vi "VisitLVType.vi"(8 "error in (no error)":errorcluster, 10 "LVType":refnum<class "LVType.lvclass">, 11 "GetTypeAttributesVisitor in":refnum<class "GetTypeAttributesVisitor.lvclass">) -> (0 "error out":errorcluster, 3 "GetTypeAttributesVisitor out":refnum<class "GetTypeAttributesVisitor.lvclass">)   [LabVIEW 2020, in "Web Service Description.lvlib" / "GetTypeAttributesVisitor.lvclass"]
uses:
  <vilib>/AppBuilder/Engine/WebServiceDescription/GetTypeAttributesVisitor/GetTypeAttributesVisitor.lvclass
  <vilib>/AppBuilder/Engine/WebServiceDescription/LVDataTypes/LVType/LVType.lvclass
  <vilib>/AppBuilder/Engine/WebServiceDescription/GetTypeAttributesVisitor/GetTypeAttributesVisitor.lvclass/GetTypeAttributesVisitor.ctl
  <vilib>/AppBuilder/Engine/WebServiceDescription/XMLGen/ValuePair.ctl
  <vilib>/AppBuilder/Engine/WebServiceDescription/XMLGen/XMLGen.lvlib
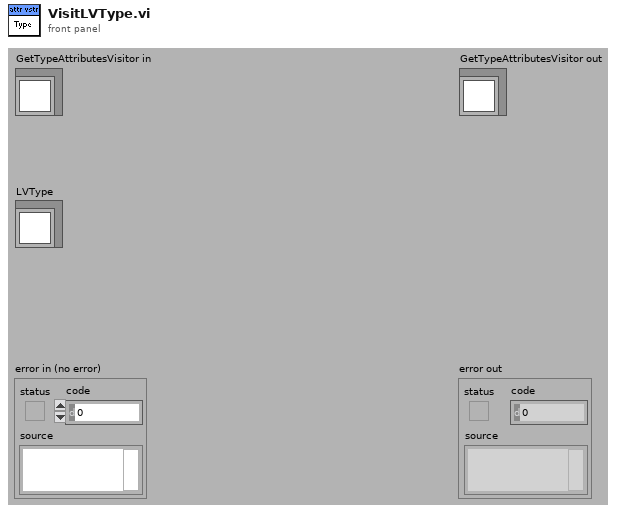
[diagram p1: front panel]
types:
  T1 = typedef "XMLGen.lvlib/ValuePair.ctl" = cluster{"Name":string, "Value":string}
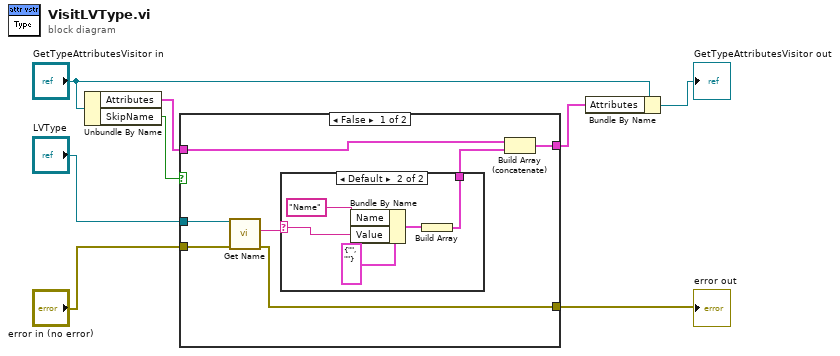
[diagram p0: block diagram]
diagram:
  n1 = Unbundle By Name("GetTypeAttributesVisitor in") -> ("Attributes"=w6:T1[], "SkipName"=w1:bool)
  n2 = case shown="False" w1 {
    tunnel: w6 -> [w15 w22]
    tunnel: "LVType" -> [w14 _]
    tunnel: "error in (no error)" -> [w13 w21]
    tunnel: [w12 w21] -> w3
    tunnel: [w11 w22] -> w2
    frame False {
      n3 = call <vilib>:"Get Name.vi"("error in (no error)"=w13, "LVType.lvclass in"=w14) -> ("error out"=w12:errorcluster, "Name"=w10:string)  [unwired: 8 out]
      n4 = case shown="Default" w10 {
        selector: w10 -> [_ w18]
        tunnel: [_ w16] -> w9
        frame "" {
        }
        frame Default {
          n5 = Bundle By Name(cluster=T1 {"Name"="", "Value"=""} ("Attribute"), "Name"="Name", "Value"=w18) -> (w17:T1)
          n6 = Build Array(w17) -> (w16:T1[])
        }
      }
      n7 = Build Array (concatenate)(w15, w9) -> (w11:T1[])
    }
    frame True {
    }
  }
  "error out" <- w3
  n8 = Bundle By Name(cluster="GetTypeAttributesVisitor in", "Attributes"=w2) -> (→"GetTypeAttributesVisitor out":refnum<class "GetTypeAttributesVisitor.lvclass">)
